vi "Ethernet Reader Modified.vi"() -> ()   [LabVIEW 2022 SP3]
doc: "This example creates a frame input stream session, reads frames at a set interval, and displays all the received frames from the latest read on the front panel."
uses:
  <vilib>/xnet/xnet.llb/XNET Frame Ethernet.ctl
  <vilib>/xnet/xnet.llb/XNET Frame Type Ethernet.ctl
  JLR/emea-tra-JLR-Synchronization-PoC/PoC_LV2020/Data.ctl
  JLR/emea-tra-JLR-Synchronization-PoC/PoC_LV2020/States.ctl
  <vilib>/userdefined/xnetEnetEptRxFilterElement.ctl
  <vilib>/xnet/xnet.llb/XNET Create Session (Frame Input Stream).vi
  <vilib>/xnet/xnet.llb/XNET Read (Frame Ethernet).vi
  <vilib>/xnet/xnet.llb/XNET Read (State Time Current).vi
  <vilib>/xnet/xnet.llb/XNET Read (State Time Trigger).vi
  <instrlib>/niSync/niSync.llb/niSync Set Time (Manual).vi
  <instrlib>/niSync/niSync.llb/niSync Initialize (Default).vi
  <resource>/objmgr/xnet.rc
panel:
  in  "CAN Cluster":refnum<k21>=":memory:"
  in  "BaudRate":u32=125000
  in  "Select Interface":refnum<k21>="CAN2"
  out "Frame Data (as hex string) Array 3":string[](array[string])
  out "Ethernet Read Frame Array 3":T1[](array[typedef]) {"fcs" format="%08x"; "network timestamp" format="%<%.7X\n%x>T"; "frame data" format="%x"; "local timestamp" format="%<%.7X\n%x>T"; "type" items=["Ethernet Data"=0, "Delay"=225, "Future Time Wait"=226]}
  in  "Generate Trigger":bool
  out "state":T3
  out "network synced 2":bool
  out "network time current 2":timestamp caption="network time current"
  out "local time current 2":timestamp caption="local time current"
  out "Port State 3":u32(ring)=3 items=["Disabled"=3, "Master"=6, "Passive"=7, "Slave"=9]
  out "Synced? 2":bool
  out "Offset From Master (ns) 2":i64
  out "Frame Data (as hex string) Array 2":string[](array[string])
  out "Ethernet Read Frame Array 2":T1[](array[typedef]) {"fcs" format="%08x"; "network timestamp" format="%<%.7X\n%x>T"; "frame data" format="%x"; "local timestamp" format="%<%.7X\n%x>T"; "type" items=["Ethernet Data"=0, "Delay"=225, "Future Time Wait"=226]}
  out "Array Size 2":i32
  out "Total Number of Frames Received 2":u64
  in  "NI Sync Resource Name 2":tag="Dev2"
  out "Time Trigger Received 2":timestamp caption="network time trigger" format="%<%.6X\n%x>T"
  in  "priority 2":u8=3
  in  "VID 2":u16=2
  in  "Interface 2":refnum<k21>="ENET1/monitor"
  out "Time Diff (Sync vs Xnet) (s)":dbl format="%#.6f"
  out "Adj Time Diff\n(Sync vs Xnet) (s)":dbl format="%#.6f"
  in  "Stop 2":bool
  out "?":T4 {"OS time set at" format="%<%.6X\n%x>T"}
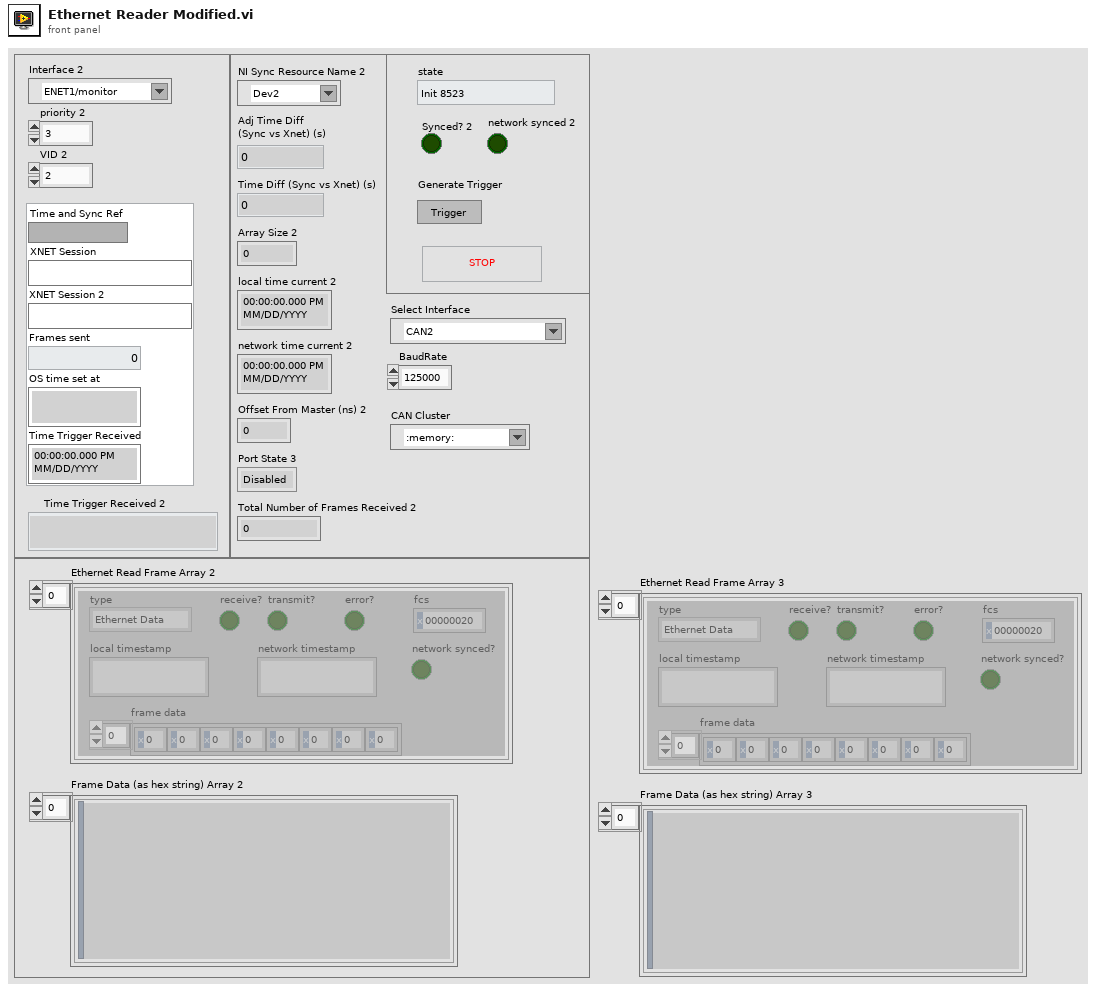
[diagram p1: front panel]
types:
  T1 = typedef "XNET Frame Ethernet.ctl" = cluster{"local timestamp":timestamp, "network timestamp":timestamp, "frame data":u8[], "fcs":u32, "type":T2, "network synced?":bool, "receive?":bool, "transmit?":bool, "error?":bool}
  T2 = typedef "XNET Frame Type Ethernet.ctl" = u16
  T3 = typedef "States.ctl" = enum16{"Init 8523", "Init 6683", "Sync 8523", "PPS+Trigger", "Set Sync Time", "Init 8510", "Adjust XNET time", "Idle", "Error"}
  T4 = typedef "Data.ctl" = cluster{"Time and Sync Ref":refnum<k15>, "XNET Session":refnum<k21>, "XNET Session 2":refnum<k21>, "Frames sent":u32, "OS time set at":timestamp, "Time Trigger Received":timestamp}
  T5 = typedef "xnetEnetEptRxFilterElement.ctl" = cluster{"use VID?":bool, "VID":u16, "use priority?":bool, "priority":u8, "use destination MAC?":bool, "destination MAC":string}
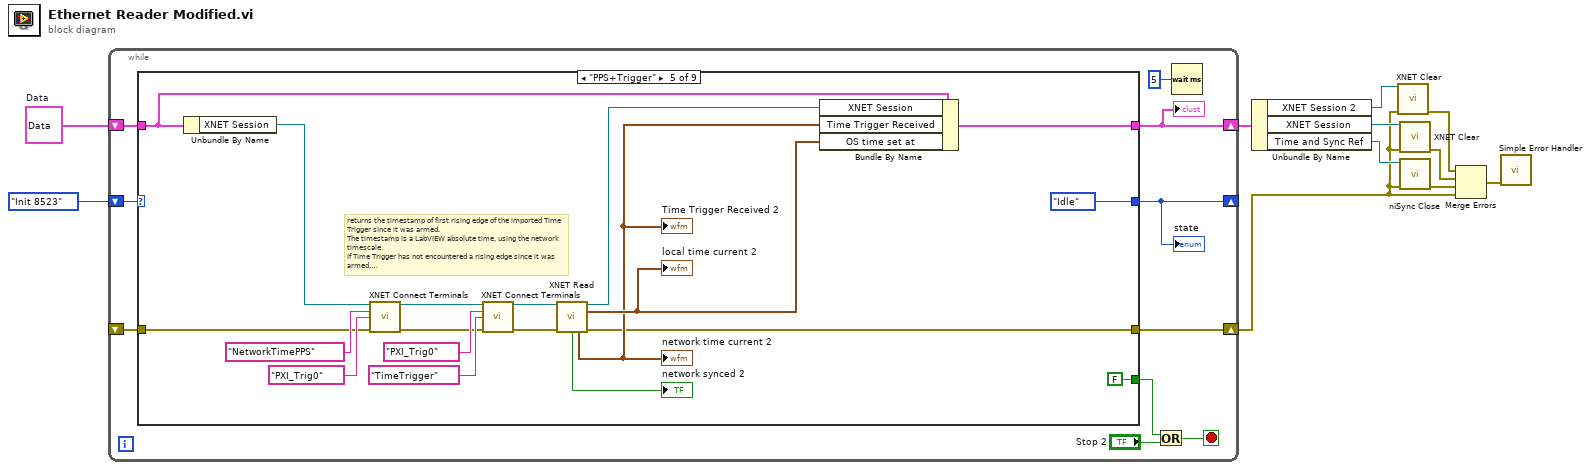
[diagram p0: block diagram]
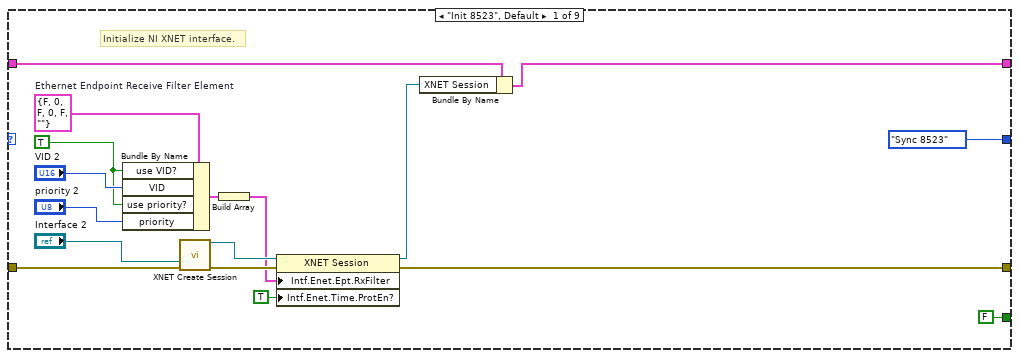
[diagram p2: hidden frame]
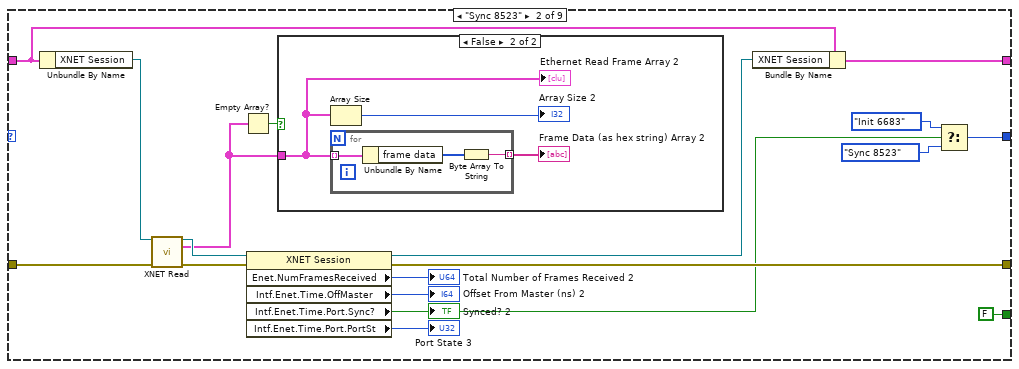
[diagram p3: hidden frame]
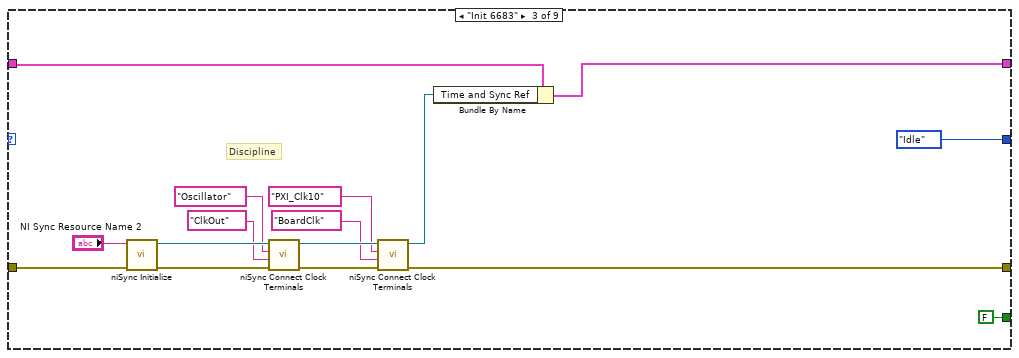
[diagram p5: hidden frame]
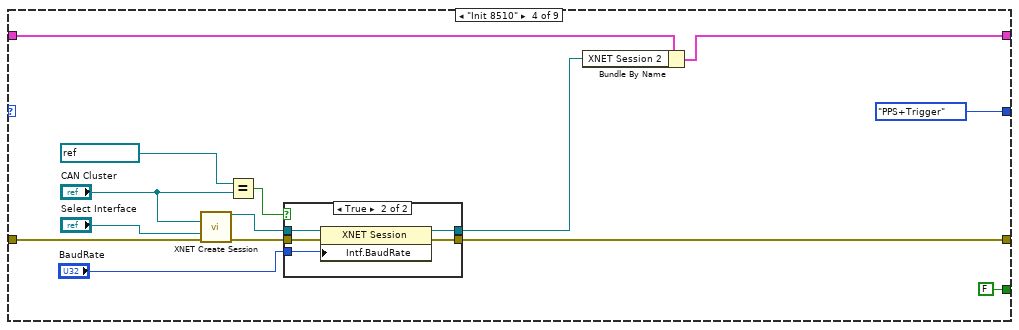
[diagram p6: hidden frame]
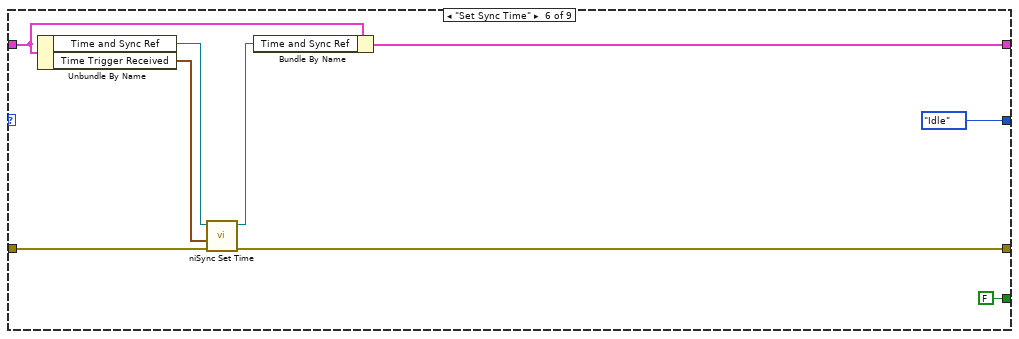
[diagram p8: hidden frame]
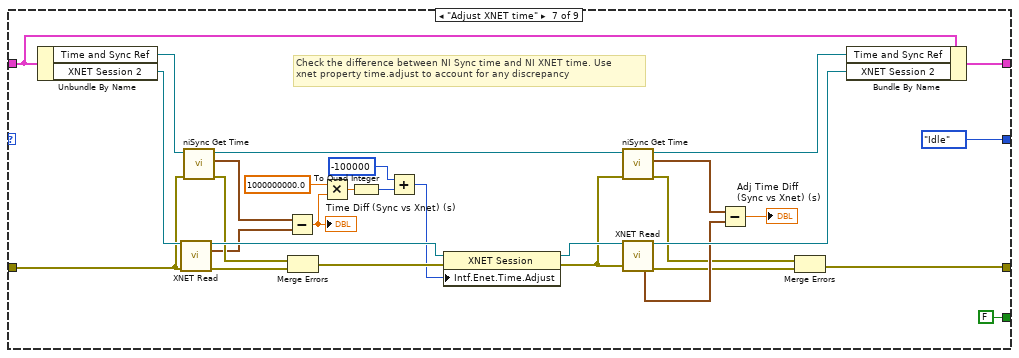
[diagram p9: hidden frame]
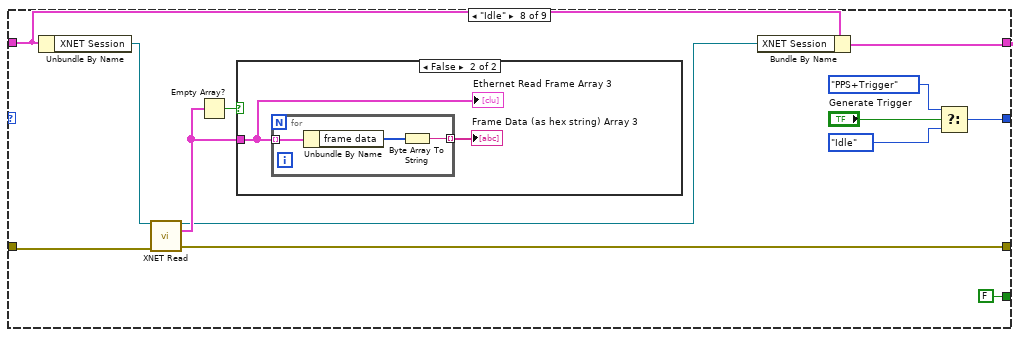
[diagram p10: hidden frame]
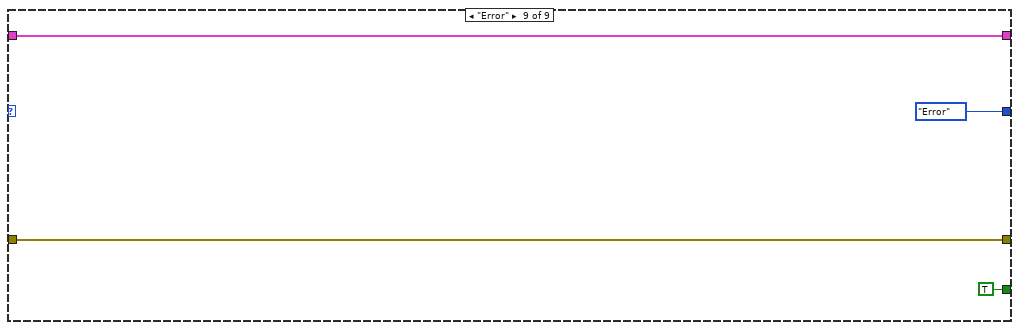
[diagram p12: hidden frame]
diagram:
  w5 = T4 {"Time and Sync Ref"="", "XNET Session"="", "XNET Session 2"="", "Frames sent"=0, "OS time set at"=timestamp(0 s since 1904-01-01), "Time Trigger Received"=timestamp(0 s since 1904-01-01)}  # Data
  n1 = while {
    shift-right: [w16] -> _
    shift-left: States."Init 8523" -> [w20]
    shift-right: [w18] -> w2
    shift-left: _ -> [w17]
    shift-right: [w13] -> w8
    shift-left: w5 -> [w19]
    stop <- w15 stop-if-true
    n2 = case shown="\"PPS+Trigger\"" w20 {
      tunnel: w19 -> [w38 w46 w69 w90 w108 w123 w130 w162 w176]
      tunnel: [w24 w52 w65 w80 w101 w121 w133 w160 w178] -> w18
      tunnel: w17 -> [w25 w43 w68 w81 w102 w125 w147 w161 w178]
      tunnel: [w36 w47 w67 w89 w107 w124 w148 w163 w176] -> w13
      tunnel: [States."Sync 8523" w49 States."Idle" States."PPS+Trigger" States."Idle" States."Idle" States."Idle" w168 States."Error"] -> w16
      tunnel: [FALSE ("Intf.Enet.Time.Port.Sync?") FALSE ("Intf.Enet.Time.Port.Sync?") FALSE ("Intf.Enet.Time.Port.Sync?") FALSE ("Intf.Enet.Time.Port.Sync?") FALSE ("Intf.Enet.Time.Port.Sync?") FALSE ("Intf.Enet.Time.Port.Sync?") FALSE ("Intf.Enet.Time.Port.Sync?") FALSE ("Intf.Enet.Time.Port.Sync?") TRUE ("Intf.Enet.Time.Port.Sync?")] -> w12
      frame "Init 8523", Default {
        w27 = TRUE ("use VID?")
        w28 = T5 {"use VID?"=FALSE, "VID"=0, "use priority?"=FALSE, "priority"=0, "use destination MAC?"=FALSE, "destination MAC"=""}  # Ethernet Endpoint Receive Filter Element
        # "Initialize NI XNET interface."
        n3 = Bundle By Name(cluster=w28, "use VID?"=w27, "VID"="VID 2", "use priority?"=w27, "priority"="priority 2") -> (w31:T5)
        n4 = call-poly <vilib>:"XNET Create Session.vi"("interface"="Interface 2", "error in (no error)"=w25) -> ("session out"=w33:refnum<k21>, "error out"=w35:errorcluster)  [unwired: 12 in]
        n5 = Build Array(w31) -> (w32:T5[])
        n6 = property class="XNET Session"(reference=w33, error in=w35, "Intf.Enet.Ept.RxFilter"=w32, "Intf.Enet.Time.ProtEn?"=TRUE ("Interface:Ethernet:Time Sync:Protocol Enabled?")) -> (reference out=w23:refnum<k21>, error out=w24:errorcluster)
        n7 = Bundle By Name(cluster=w38, "XNET Session"=w23) -> (w36:T4)
      }
      frame "Sync 8523" {
        n8 = Unbundle By Name(w46) -> ("XNET Session"=w45:refnum<k21>)
        n9 = call-poly <vilib>:"XNET Read.vi"("session in"=w45, "error in (no error)"=w43) -> ("session out"=w42:refnum<k21>, "data"=w41:T1[], "error out"=w44:errorcluster)  [unwired: 10 in, 1 out]
        n10 = Empty Array?(array=w41) -> (empty?=w55:bool)
        n11 = property class="XNET Session"(reference=w42, error in=w44) -> (reference out=w48:refnum<k21>, error out=w52:errorcluster, "Enet.NumFramesReceived"=→"Total Number of Frames Received 2":u64, "Intf.Enet.Time.OffMaster"=→"Offset From Master (ns) 2":i64, "Intf.Enet.Time.Port.Sync?"=w40:bool, "Intf.Enet.Time.Port.PortSt"=→"Port State 3":u32)
        "Synced? 2" <- w40
        n12 = case shown="False" w55 {
          tunnel: w41 -> [_ w57]
          frame True {
          }
          frame False {
            n13 = Array Size(array=w57) -> (size(s)=→"Array Size 2":i32)
            n14 = for {
              tunnel: [w62] -> w59 mode=indexing
              tunnel: w57 -> [w61] mode=indexing
              n15 = Unbundle By Name(w61) -> ("frame data"=w60:u8[])
              n16 = Byte Array To String(unsigned byte array=w60) -> (string=w62:string)
            }
            "Frame Data (as hex string) Array 2" <- w59
            "Ethernet Read Frame Array 2" <- w57
          }
        }
        n17 = Bundle By Name(cluster=w46, "XNET Session"=w48) -> (w47:T4)
        n18 = Select(t=States."Init 6683", s=w40, f=States."Sync 8523") -> (s? t:f=w49:T3)
      }
      frame "Init 6683" {
        # "Discipline"
        n19 = call-poly <instrlib>:"niSync Initialize.vi"("error in (no error)"=w68, "resource name"="NI Sync Resource Name 2") -> ("error out"=w78:errorcluster, "instrument handle out"=w77:refnum<k15>)  [unwired: 8 in]
        n20 = call <instrlib>:"niSync Connect Clock Terminals.vi"("error in (no error)"=w78, "destination terminal"="ClkOut", "source terminal"="Oscillator", "instrument handle"=w77) -> ("error out"=w75:errorcluster, "instrument handle out"=w76:refnum<k15>)  [unwired: 6 in]
        n21 = call <instrlib>:"niSync Connect Clock Terminals.vi"("error in (no error)"=w75, "destination terminal"="BoardClk", "source terminal"="PXI_Clk10", "instrument handle"=w76) -> ("error out"=w65:errorcluster, "instrument handle out"=w64:refnum<k15>)  [unwired: 6 in]
        n22 = Bundle By Name(cluster=w69, "Time and Sync Ref"=w64) -> (w67:T4)
      }
      frame "Init 8510" {
        n23 = call-poly <vilib>:"XNET Create Session.vi"("cluster (:memory:)"="CAN Cluster", "interface"="Select Interface", "error in (no error)"=w81) -> ("session out"=w87:refnum<k21>, "error out"=w85:errorcluster)  [unwired: 11 out]
        n24 = Equal?(x=refnum<k21> ":memory:" ("CAN Cluster"), y="CAN Cluster") -> (x = y?=w84:bool)
        n25 = case shown="True" w84 {
          tunnel: w87 -> [w94 w99]
          tunnel: [w94 w98] -> w79
          tunnel: "BaudRate" -> [_ w97]
          tunnel: [w93 w96] -> w80
          tunnel: w85 -> [w93 w95]
          frame False {
          }
          frame True {
            n26 = property class="XNET Session"(reference=w99, error in=w95, "Intf.BaudRate"=w97) -> (reference out=w98:refnum<k21>, error out=w96:errorcluster)
          }
        }
        n27 = Bundle By Name(cluster=w90, "XNET Session 2"=w79) -> (w89:T4)
      }
      frame "PPS+Trigger" {
        # "returns the timestamp of first rising edge of the imported Time Trigger since it was armed. \nThe timestamp is a LabVIEW absolute time, using the network timescale. \nIf Time Trigger has not encountered a rising edge since it was armed, \nnetwork time trigger returns zero (an invalid timestamp)."
        n28 = Unbundle By Name(w108) -> ("XNET Session"=w110:refnum<k21>)
        n29 = call <vilib>:"XNET Connect Terminals.vi"("session in"=w110, "source terminal"=tag "NetworkTimePPS", "destination terminal"=tag "PXI_Trig0", "error in (no error)"=w102) -> ("session out"=w113:refnum<k21>, "error out"=w114:errorcluster)  [unwired: 10 in]
        n30 = call <vilib>:"XNET Connect Terminals.vi"("session in"=w113, "source terminal"=tag "PXI_Trig0", "destination terminal"=tag "TimeTrigger", "error in (no error)"=w114) -> ("session out"=w109:refnum<k21>, "error out"=w111:errorcluster)  [unwired: 10 in]
        n31 = call-poly <vilib>:"XNET Read.vi"("session in"=w109, "error in (no error)"=w111) -> ("session out"=w118:refnum<k21>, "local time trigger"=w104:timestamp, "network synced"=→"network synced 2":bool, "network time trigger"=w103:timestamp, "error out"=w101:errorcluster)  [unwired: 9 in]
        "Time Trigger Received 2" <- w103
        "local time current 2" <- w104
        "network time current 2" <- w103
        n32 = Bundle By Name(cluster=w108, "XNET Session"=w118, "Time Trigger Received"=w103, "OS time set at"=w104) -> (w107:T4)
      }
      frame "Set Sync Time" {
        n33 = Unbundle By Name(w123) -> ("Time and Sync Ref"=w126:refnum<k15>, "Time Trigger Received"=w122:timestamp)
        n34 = call-poly <instrlib>:"niSync Set Time.vi"("error in (no error)"=w125, "initial time"=w122, "instrument handle"=w126) -> ("error out"=w121:errorcluster, "instrument handle out"=w120:refnum<k15>)  [unwired: 7 in]
        n35 = Bundle By Name(cluster=w123, "Time and Sync Ref"=w120) -> (w124:T4)
      }
      frame "Adjust XNET time" {
        # "Check the difference between NI Sync time and NI XNET time. Use\nxnet property time.adjust to account for any discrepancy"
        n36 = Unbundle By Name(w130) -> ("Time and Sync Ref"=w149:refnum<k15>, "XNET Session 2"=w150:refnum<k21>)
        n37 = call-poly <vilib>:"XNET Read.vi"("session in"=w150, "error in (no error)"=w147) -> ("session out"=w152:refnum<k21>, "local time current"=w129:timestamp, "error out"=w151:errorcluster)  [unwired: 9 in, 2 out]
        n38 = call <instrlib>:"niSync Get Time.vi"("error in (no error)"=w147, "instrument handle"=w149) -> ("error out"=w145:errorcluster, "time"=w157:timestamp, "instrument handle out"=w141:refnum<k15>)  [unwired: 5 in]
        n39 = Subtract(x=w157, y=w129) -> (x-y=w156:dbl)
        "Time Diff (Sync vs Xnet) (s)" <- w156
        n40 = Merge Errors(w145, w151) -> (w146:errorcluster)
        n41 = Multiply(x=1000000000.0 ("y"), y=w156) -> (x*y=w154:dbl)
        n42 = To Quad Integer(1:w154) -> (0:w153:i64)
        n43 = Add(x=i64 -100000, y=w153) -> (x+y=w132:i64)
        n44 = property class="XNET Session"(reference=w152, error in=w146, "Intf.Enet.Time.Adjust"=w132) -> (reference out=w143:refnum<k21>, error out=w140:errorcluster)
        n45 = call <instrlib>:"niSync Get Time.vi"("error in (no error)"=w140, "instrument handle"=w141) -> ("error out"=w134:errorcluster, "time"=w138:timestamp, "instrument handle out"=w137:refnum<k15>)  [unwired: 5 in]
        n46 = call-poly <vilib>:"XNET Read.vi"("session in"=w143, "error in (no error)"=w140) -> ("session out"=w142:refnum<k21>, "network time current"=w136:timestamp, "error out"=w135:errorcluster)  [unwired: 9 in, 2 out]
        n47 = Subtract(x=w138, y=w136) -> (x-y=→"Adj Time Diff\n(Sync vs Xnet) (s)":dbl)
        n48 = Merge Errors(w134, w135) -> (w133:errorcluster)
        n49 = Bundle By Name(cluster=w130, "Time and Sync Ref"=w137, "XNET Session 2"=w142) -> (w148:T4)
      }
      frame "Idle" {
        n50 = Unbundle By Name(w162) -> ("XNET Session"=w165:refnum<k21>)
        n51 = call-poly <vilib>:"XNET Read.vi"("session in"=w165, "error in (no error)"=w161) -> ("session out"=w159:refnum<k21>, "data"=w164:T1[], "error out"=w160:errorcluster)  [unwired: 10 in, 1 out]
        n52 = Empty Array?(array=w164) -> (empty?=w166:bool)
        n53 = case shown="False" w166 {
          tunnel: w164 -> [_ w171]
          frame True {
          }
          frame False {
            n54 = for {
              tunnel: [w175] -> w172 mode=indexing
              tunnel: w171 -> [w174] mode=indexing
              n55 = Unbundle By Name(w174) -> ("frame data"=w173:u8[])
              n56 = Byte Array To String(unsigned byte array=w173) -> (string=w175:string)
            }
            "Frame Data (as hex string) Array 3" <- w172
            "Ethernet Read Frame Array 3" <- w171
          }
        }
        n57 = Bundle By Name(cluster=w162, "XNET Session"=w159) -> (w163:T4)
        n58 = Select(t=States."PPS+Trigger", s="Generate Trigger", f=States."Idle") -> (s? t:f=w168:T3)
      }
      frame "Error" {
      }
    }
    "?" <- w13
    "state" <- w16
    n59 = Or(x=w12, y="Stop 2") -> (x .or. y?=w15:bool)
    n60 = Wait (ms)(milliseconds to wait=u32 5) -> ()  [unwired: 1 out]
  }
  n61 = Unbundle By Name(w8) -> ("XNET Session 2"=w3:refnum<k21>, "XNET Session"=w7:refnum<k21>, "Time and Sync Ref"=w6:refnum<k15>)
  n62 = call <vilib>:"XNET Clear.vi"("session in"=w3, "error in (no error)"=w2) -> ("error out"=w1:errorcluster)  [unwired: 13 in]
  n63 = call <vilib>:"XNET Clear.vi"("session in"=w7, "error in (no error)"=w2) -> ("error out"=w11:errorcluster)  [unwired: 13 in]
  n64 = call <instrlib>:"niSync Close.vi"("error in (no error)"=w2, "instrument handle"=w6) -> ("error out"=w9:errorcluster)  [unwired: 9 in]
  n65 = Merge Errors(w1, w11, w9, w2) -> (w10:errorcluster)
  n66 = call <vilib>:"Simple Error Handler.vi"("error in (no error)"=w10) -> ()  [unwired: 4 in, 5 out]
